vi "micron_update.vi"(0 "Position valid":bool, 2 "XYZ in":sgl[][](array[numeric])=[[-1290.5378, -2714.2402, -42.909184], [-1227.3542, -3608.3708, 102.94437]] format="%#.2f", 5 "Micron config":T12, 6 "error in":errorcluster, 8 "No pose":bool, 10 "Reset":bool, 11 "Trace index":i32, 16 "Parameters":T1={"Stimulus"={"Type"=enum."Off", "Phase"=0.0, "Amplitude"=[], "Injection point"=enum."Total pose", "Closed loop"=FALSE, "Offset"=[], "Tip -> world"=FALSE, "Frequency"=0.0, "Length"=0.0}, "Goal Filter A"={"Speedup max"=0.0, "Speedup thresh"=0.0, "Speedup nonlin"=0.0, "Filters"=[]}, "Mode controls"={"Hold"=FALSE, "Cancellation"=FALSE, "Goal filter"=FALSE, "Trigger"=FALSE}, "Manipulator type"=enum."Current piezo", "Manipulator calibration"={"Tool offsets"=[[0.0, 0.0, 36200.0]], "Handle light calibration"=[], "Base pivots"=[], "Output pivots"=[], "Length center"=0.0, "Workspace height"=[], "Workspace diameter"=[0.0, 0.0, 36200.0], "Stack travel"=400.0, "Saturation pos"=375.0, "Inverse filters"=[], "Strut length"=0.0, "Tip light calibration"=[]}, "Network"={"Remote Host"="", "Send Status"=FALSE, "Send Port"=0, "Recv Commands"=FALSE, "Recv Port"=0}, "Goal Filter B"={"Speedup max"=0.0, "Speedup thresh"=0.0, "Speedup nonlin"=0.0, "Filters"=[]}, "Cancellation"={"KP"={"XY"=0.0, "Rxy"=0.0, "Z"=0.0, "Rz"=0.0}, "KI"=0.0, "KD"={"XY"=0.0, "Rxy"=0.0, "Z"=0.0, "Rz"=0.0}, "Max vel"=20.0, "Max acc"=0.001, "Int error limit"=3.0, "RCM gain"=0.0, "Bypass"=FALSE, "Degraded gain"=0.0}, "Transition time"=0.0, "Estimation"={"Link"={"Measure noise"=[], "Process noise"=[], "Alt process noise"=[], "Alt turnoff cycles"=20, "Innovation limit"=[], "Residue threshold"=0.0, "Enable"=FALSE}, "Handle"={"Measure noise"=[], "Process noise"=[], "State limits"=[], "Innovation limit"=[], "Prediction Lookahead"=0.0, "Enable"=FALSE}}} {"Transition time" format="%_3f"; "Cancellation"."Degraded gain" min=0 max=1 step=0.1 format="%#_3p"; "Cancellation"."RCM gain" min=0 max=1 step=0.1 format="%#_3p"; "Cancellation"."KD"."Rz" min=-1 max=1 step=0.01 format="%#_3p"; "Cancellation"."KD"."Rxy" min=-1 max=1 step=0.01 format="%#_3p"; "Cancellation"."KD"."Z" min=-1 max=1 step=0.01 format="%#_3p"; "Cancellation"."KD"."XY" min=-1 max=1 step=0.01 format="%#_3p"; "Cancellation"."KI" min=0 max=1 step=0.01 format="%#_3p"; "Cancellation"."KP"."Rz" min=-1 max=1 step=0.01 format="%#_3p"; "Cancellation"."KP"."Rxy" min=-1 max=1 step=0.01 format="%#_3p"; "Cancellation"."KP"."Z" min=-1 max=1 step=0.01 format="%#_3p"; "Cancellation"."KP"."XY" min=-1 max=1 step=0.01 format="%#_3p"; "Cancellation"."Max acc" format="%#_3p"; "Goal Filter B"."Filters"."V limit range" format="%_3p"; "Goal Filter B"."Filters"."V limit" format="%_3p"; "Goal Filter B"."Filters"."Upper Q" format="%_3f"; "Goal Filter B"."Filters"."Upper Fc" format="%_3p"; "Goal Filter B"."Filters"."Lower Q" format="%_3f"; "Goal Filter B"."Filters"."Scale factor" format="%_3f"; "Goal Filter B"."Filters"."Lower Fc" format="%_3p"; "Goal Filter B"."Speedup nonlin" format="%_3p"; "Goal Filter B"."Speedup thresh" format="%_3p"; "Goal Filter B"."Speedup max" format="%_3p"; "Manipulator calibration"."Tip light calibration" format="%#.1f"; "Manipulator calibration"."Strut length" format="%#_4p"; "Manipulator calibration"."Saturation pos" format="%#.1f"; "Manipulator calibration"."Stack travel" format="%#.1f"; "Manipulator calibration"."Length center" format="%#_4p"; "Manipulator calibration"."Output pivots" format="%#_6f"; "Manipulator calibration"."Base pivots" format="%#_6f"; "Manipulator calibration"."Handle light calibration" format="%#.1f"; "Goal Filter A"."Filters"."V limit range" format="%_3p"; "Goal Filter A"."Filters"."V limit" format="%_3p"; "Goal Filter A"."Filters"."Upper Q" format="%_3f"; "Goal Filter A"."Filters"."Upper Fc" format="%_3p"; "Goal Filter A"."Filters"."Lower Q" format="%_3f"; "Goal Filter A"."Filters"."Scale factor" format="%_3f"; "Goal Filter A"."Filters"."Lower Fc" format="%_3p"; "Goal Filter A"."Speedup nonlin" format="%_3p"; "Goal Filter A"."Speedup thresh" format="%_3p"; "Goal Filter A"."Speedup max" format="%_3p"; "Stimulus"."Length" min=0.0 max=100.0 step=100.0 format="%#_4p"; "Stimulus"."Frequency" min=0.0 step=100.0 format="%#_4g"; "Stimulus"."Offset" format="%#_3p"; "Stimulus"."Amplitude" format="%#_3p"; "Stimulus"."Phase" min=-180.0 max=360.0 step=100.0 format="%#.2f"}) -> (17 "Timestamp":u64, 26 "error out":errorcluster)   [LabVIEW 2014]
uses:
  initialization/micron_config.ctl
  manipulator/squiggle/Host/i2c_interface.ctl
  manipulator/squiggle/Host/fpga_reference.ctl
  testing/Micron params.ctl
  testing/stimulus.ctl
  testing/injection_point.ctl
  filtering/goal_loop_parms.ctl
  testing/mode_conrols.ctl
  testing/manipulator_cal.ctl
  asap/labview/testing/probe_calibration.ctl
  host/network_params.ctl
  sq_control_params.ctl
  decoupled_gain.ctl
  estimation_controls.ctl
  <vilib>/Analysis/Matrix/Datatypes/RealMatrix.ctl
  initialization/micron_globals.vi
  <vilib>/Analysis/Matrix/Numeric/Conversions/Matrix To Array - RM.vi
  <vilib>/Analysis/Matrix/NI_Matrix.lvlib
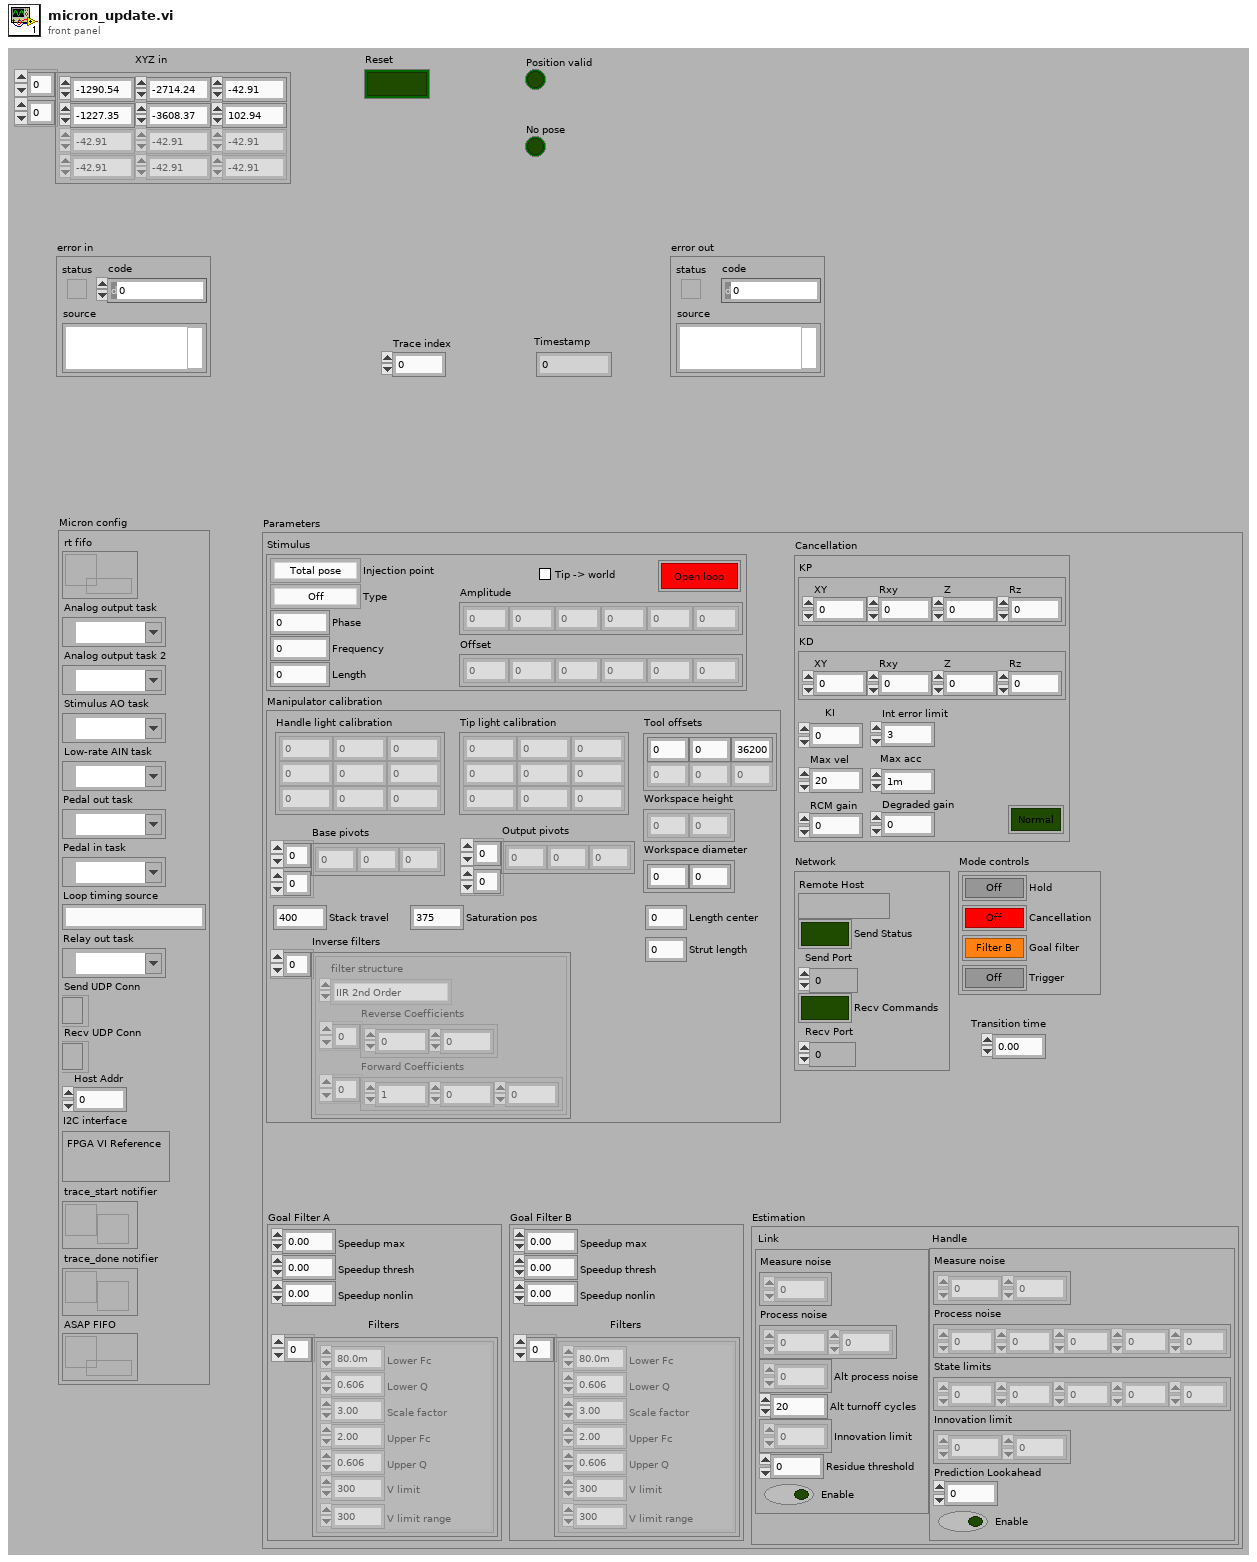
[diagram p1: front panel]
types:
  T1 = typedef "Micron params.ctl" = cluster{"Stimulus":T2, "Goal Filter A":T4, "Mode controls":T5, "Manipulator type":enum16{"Current piezo", "Voltage piezo"}, "Manipulator calibration":T6, "Network":T8, "Goal Filter B":T4, "Cancellation":T9, "Transition time":sgl, "Estimation":T11}
  T2 = typedef "stimulus.ctl" = cluster{"Type":enum16{"Off", "Step", "Sine", "Triangle", "Arbitrary"}, "Phase":dbl, "Amplitude":sgl[], "Injection point":T3, "Closed loop":bool, "Offset":sgl[], "Tip -> world":bool, "Frequency":dbl, "Length":dbl}
  T3 = typedef "injection_point.ctl" = enum16{"Total pose", "V limiter", "Goal ", "Link position", "KF link position", "Inverse kin", "Link goal", "Link error", "Controller", "Output", "Drive", "Light"}
  T4 = typedef "goal_loop_parms.ctl" = cluster{"Speedup max":sgl, "Speedup thresh":sgl, "Speedup nonlin":sgl, "Filters":cluster{"Lower Fc":sgl, "Lower Q":sgl, "Scale factor":sgl, "Upper Fc":sgl, "Upper Q":sgl, "V limit":sgl, "V limit range":sgl}[]}
  T5 = typedef "mode_conrols.ctl" = cluster{"Hold":bool, "Cancellation":bool, "Goal filter":bool, "Trigger":bool}
  T6 = typedef "manipulator_cal.ctl" = cluster{"Tool offsets":sgl[][], "Handle light calibration":T7, "Base pivots":sgl[][], "Output pivots":sgl[][], "Length center":sgl, "Workspace height":sgl[], "Workspace diameter":sgl[], "Stack travel":sgl, "Saturation pos":sgl, "Inverse filters":cluster{"filter structure":enum32{"IIR 2nd Order", "IIR 4th Order"}, "Reverse Coefficients":dbl[], "Forward Coefficients":dbl[]}[], "Strut length":sgl, "Tip light calibration":T7}
  T7 = typedef "probe_calibration.ctl" = sgl[][]
  T8 = typedef "network_params.ctl" = cluster{"Remote Host":string, "Send Status":bool, "Send Port":u16, "Recv Commands":bool, "Recv Port":u16}
  T9 = typedef "sq_control_params.ctl" = cluster{"KP":T10, "KI":sgl, "KD":T10, "Max vel":sgl, "Max acc":sgl, "Int error limit":sgl, "RCM gain":sgl, "Bypass":bool, "Degraded gain":sgl}
  T10 = typedef "decoupled_gain.ctl" = cluster{"XY":sgl, "Rxy":sgl, "Z":sgl, "Rz":sgl}
  T11 = typedef "estimation_controls.ctl" = cluster{"Link":cluster{"Measure noise":dbl[], "Process noise":dbl[], "Alt process noise":dbl[], "Alt turnoff cycles":i32, "Innovation limit":dbl[], "Residue threshold":dbl, "Enable":bool}, "Handle":cluster{"Measure noise":dbl[], "Process noise":dbl[], "State limits":dbl[], "Innovation limit":dbl[], "Prediction Lookahead":sgl, "Enable":bool}}
  T12 = typedef "micron_config.ctl" = cluster{"rt fifo":refnum<k33>, "Analog output task":refnum<k21>, "Analog output task 2":refnum<k21>, "Stimulus AO task":refnum<k21>, "Low-rate AIN task":refnum<k21>, "Pedal out task":refnum<k21>, "Pedal in task":refnum<k21>, "Loop timing source":string, "Relay out task":refnum<k21>, "Send UDP Conn":refnum<k16>, "Recv UDP Conn":refnum<k16>, "Host Addr":u32, "I2C interface":T13, "trace_start notifier":refnum<notifier>, "trace_done notifier":refnum<notifier>, "ASAP FIFO":refnum<k33>}
  T13 = typedef "i2c_interface.ctl" = cluster{"FPGA VI Reference":T14}
  T14 = typedef "fpga_reference.ctl" = refnum<k20>
  T15 = typedef "NI_Matrix.lvlib/RealMatrix.ctl" = dbl[][]
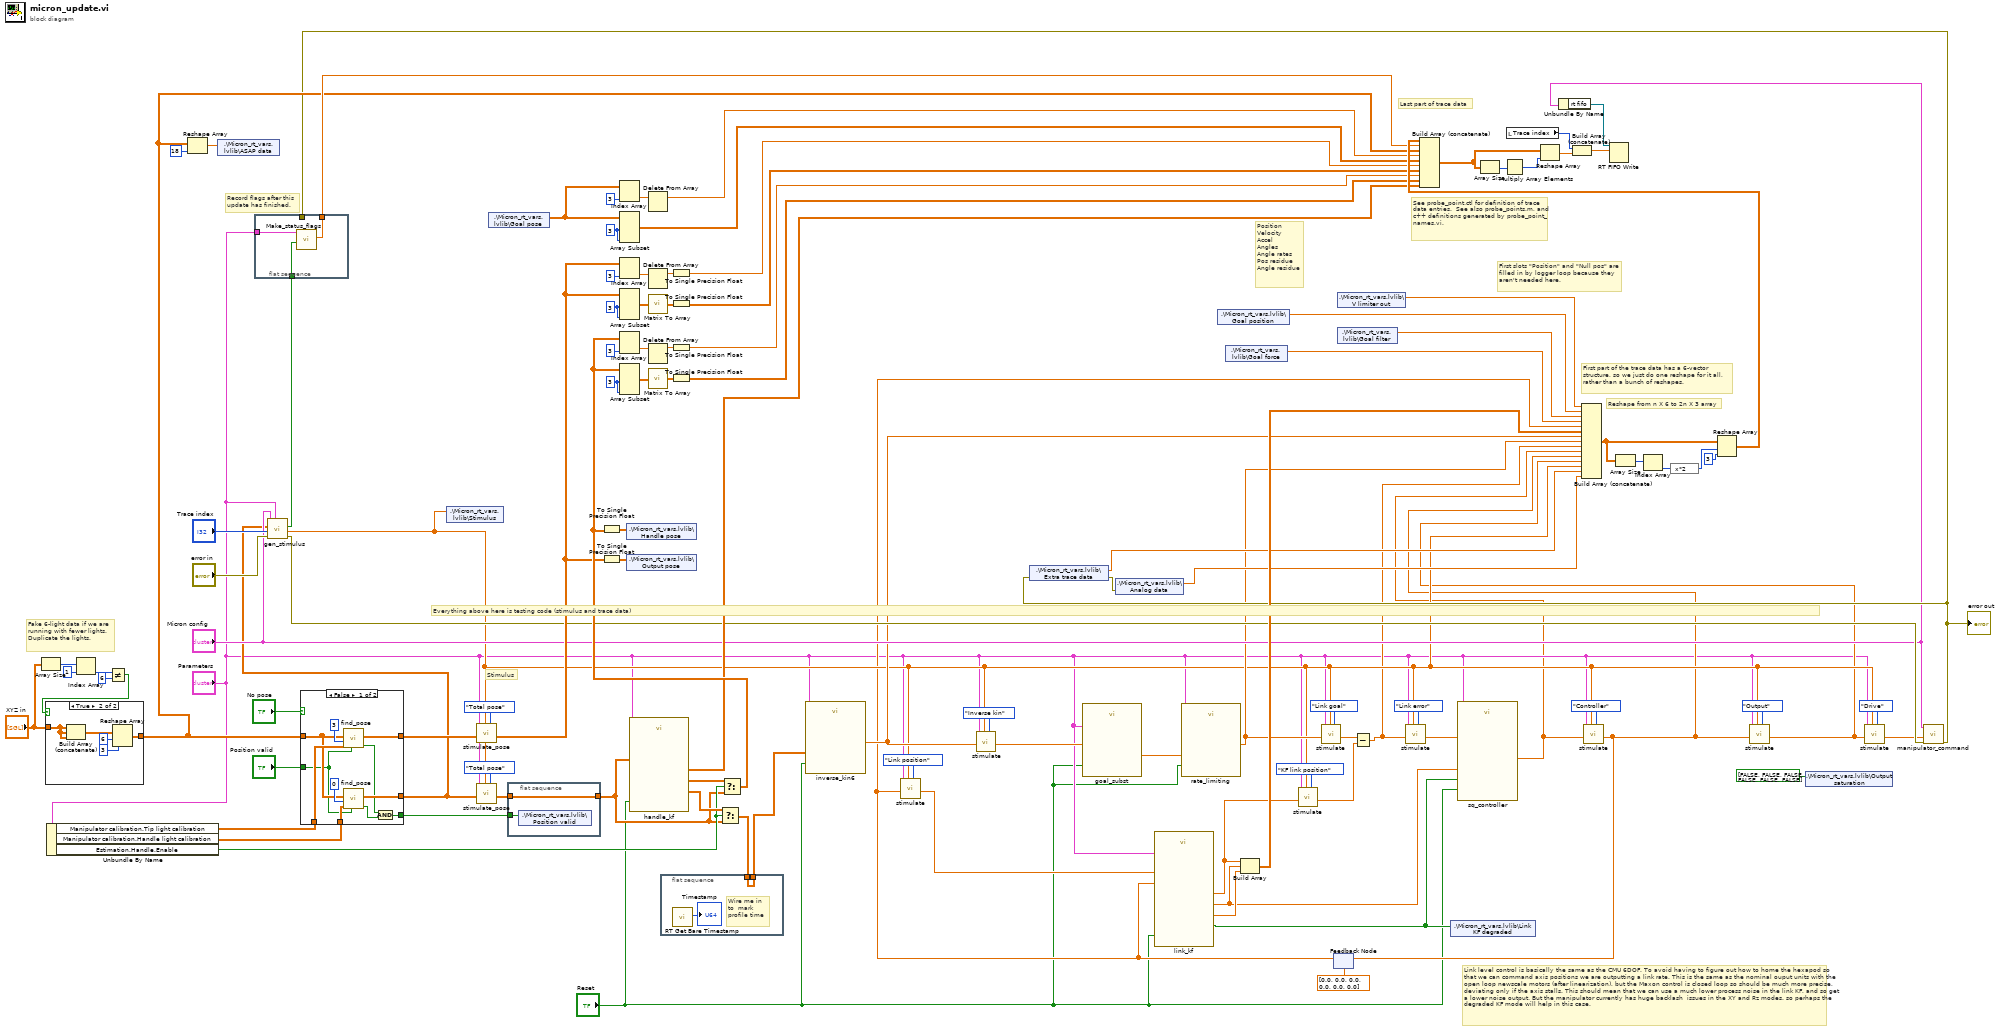
[diagram p0: block diagram]
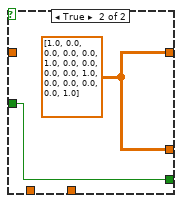
[diagram p2: hidden frame]
diagram:
  w73 = 3 ("length")
  w80 = 3 ("length")
  w107 = 3 ("length")
  # "Link level control is basically the same as the CMU 6DOF. To avoid having to figure out how to home the hexapod so that we can command axis positions we are outputting a link rate. This is the same as the nominal ouput units with the open loop newscale motors (after linearization), but the Maxon control is closed loop so should be much more precise, deviating only if the axis stalls. This should mean that we can use a much lower process noise in the link KF, and so get a lower noise output. But the manipulator currently has huge backlash  issues in the XY and Rz modes. so perhaps the degraded KF mode will help in this case."
  # "Position\nVelocity\nAccel\nAngles\nAngle rates\nPos residue\nAngle residue"
  # "Record flags after this\nupdate has finished."
  # "Fake 6-light data if we are running with fewer lights. Duplicate the lights."
  # "First slots \"Position\" and \"Null pos\" are filled in by logger loop because they aren't needed here."
  # "Last part of trace data"
  # "First part of the trace data has a 6-vector structure, so we just do one reshape for it all, rather than a bunch of reshapes."
  # "Reshape from n X 6 to 2n X 3 array"
  # "Everything above here is testing code (stimulus and trace data)"
  # "Stimulus"
  # "See probe_point.ctl for definition of trace data entries.  See also probe_points.m, and c++ definitions generated by probe_point_names.vi."
  n1 = Array Size(array="XYZ in") -> (size(s)=w51:i32[])
  n2 = Unbundle By Name("Parameters") -> ("Manipulator calibration.Tip light calibration"=w86:T7, "Manipulator calibration.Handle light calibration"=w67:T7, "Estimation.Handle.Enable"=w57:bool)
  n3 = Index Array(array=w51, index=1) -> (element=w49:i32)
  n4 = Not Equal?(x=w49, y=6) -> (x != y?=w47:bool)
  n5 = case shown="True" w47 {
    tunnel: [w112 w115] -> w64
    tunnel: "XYZ in" -> [w112 w113]
    frame False {
    }
    frame True {
      n6 = Build Array (concatenate)(w113, w113, w113) -> (w114:sgl[][])
      n7 = Reshape Array(w114, 6 ("dimension size"), 3 ("dimension size")) -> (w115:sgl[][])
    }
  }
  n8 = Reshape Array(w64, 18 ("dimension size")) -> (w101:sgl[])
  n9 = shared-variable ".\\Micron_rt_vars.lvlib\\ASAP data"(w101) -> ()  [unwired: 2 out]
  n10 = flat-sequence {
    tunnel: [w120] -> w88
    tunnel: w56 -> [w119]
    tunnel: "Parameters" -> [w118]
    tunnel: w44 -> [_]
    frame #0 {
      n11 = call "Make_status_flags.vi"("Stimulus increasing"=w119, "Parameters"=w118) -> ("Status flags"=w120:sgl[])  [unwired: 9 out]
    }
  }
  n12 = case shown="False" "No pose" {
    tunnel: w86 -> [w130 _]
    tunnel: w67 -> [w129 _]
    tunnel: w64 -> [w127 _]
    tunnel: [w126 w132] -> w63
    tunnel: [w125 w132] -> w30
    tunnel: "Position valid" -> [w124 w133]
    tunnel: [w121 w133] -> w17
    frame False {
      n13 = call "find_pose.vi"("Position valid"=w124, "Light positions"=w130, "XYZ index"=3, "XYZ in"=w127) -> ("Pose valid"=w123:bool, "Pose"=w126:T15)  [unwired: 1 in, 5 out]
      n14 = call "find_pose.vi"("Position valid"=w124, "Light positions"=w129, "XYZ index"=0, "XYZ in"=w127) -> ("Pose valid"=w122:bool, "Pose"=w125:T15)  [unwired: 1 in, 5 out]
      n15 = And(x=w123, y=w122) -> (x .and. y?=w121:bool)
    }
    frame True {
      w132 = T15 [[1.0, 0.0, 0.0, 0.0], [0.0, 1.0, 0.0, 0.0], [0.0, 0.0, 1.0, 0.0], [0.0, 0.0, 0.0, 1.0]] ("LR transform")
    }
  }
  n16 = call "gen_stimulus.vi"("Parameters"="Parameters", "error in"="error in", "Trace index"="Trace index", "Raw handle pose"=w30, "Micron config"="Micron config") -> ("error out"=w55:errorcluster, "Stimulus"=w22:sgl[], "Stimulus increasing"=w56:bool)  [unwired: 4 out]
  n17 = shared-variable ".\\Micron_rt_vars.lvlib\\Stimulus"(w22) -> ()  [unwired: 2 out]
  n18 = call "stimulate_pose.vi"("Injection point"=injection_point."Total pose", "Stimulus"=w22, "Pose in"=w63, "Parameters"="Parameters") -> ("Pose out"=w61:T15)  [unwired: 6 in]
  n19 = call "stimulate_pose.vi"("Injection point"=injection_point."Total pose", "Stimulus"=w22, "Pose in"=w30, "Parameters"="Parameters") -> ("Pose out"=w19:T15)  [unwired: 6 in]
  n20 = shared-variable ".\\Micron_rt_vars.lvlib\\Goal pose"() -> (w70:sgl[][])  [unwired: 2 out]
  n21 = flat-sequence {
    tunnel: [w135] -> w18
    tunnel: w19 -> [w135]
    tunnel: w17 -> [w134]
    frame #0 {
      n22 = shared-variable ".\\Micron_rt_vars.lvlib\\Position valid"(w134) -> ()  [unwired: 2 out]
    }
  }
  n23 = To Single Precision Float(number=w61) -> (single precision float=w102:sgl[][])
  n24 = Index Array(array=w70, index (col)=3 ("disabled index (col)")) -> (element=w72:sgl[])  [unwired: 1 in]
  n25 = Array Subset(array=w70, length (row)=w73, length (col)=w73) -> (w69:sgl[][])  [unwired: 2 in]
  n26 = Index Array(array=w61, index (col)=3 ("disabled index (col)")) -> (element=w99:dbl[])  [unwired: 1 in]
  n27 = Array Subset(array=w61, length (row)=w107, length (col)=w107) -> (w106:T15)  [unwired: 2 in]
  n28 = shared-variable ".\\Micron_rt_vars.lvlib\\Output pose"(w102) -> ()  [unwired: 2 out]
  n29 = call "handle_kf.vi"("Reset"="Reset", "Parameters"="Parameters", "Handle Pose"=w18) -> ("Handle State"=w65:sgl[][], "Predicted Handle Pose"=w58:T15, "Handle Pose (KF)"=w59:T15)  [unwired: 6 in]
  n30 = Delete From Array(array=w72) -> (array with subset deleted=w26:sgl[])  [unwired: 2 in, 1 out]
  n31 = Delete From Array(array=w99) -> (array with subset deleted=w97:dbl[])  [unwired: 2 in, 1 out]
  n32 = call-poly <vilib>:"Matrix To Array.vi"("Real Matrix"=w106) -> ("Real 2D Array"=w105:dbl[][])
  n33 = flat-sequence {
    tunnel: [w136] -> w53
    tunnel: w54 -> [w136]
    frame #0 {
      # "Wire me in to  mark profile time"
      n34 = call "RT Get Bare Timestamp.vi"() -> ("Timestamp"=→"Timestamp":u64)  [unwired: 11 out]
    }
  }
  n35 = To Single Precision Float(number=w97) -> (single precision float=w25:sgl[])
  n36 = To Single Precision Float(number=w105) -> (single precision float=w89:sgl[][])
  n37 = Select(t=w58, s=w57, f=w18) -> (s? t:f=w54:T15)
  n38 = Select(t=w59, s=w57, f=w18) -> (s? t:f=w66:T15)
  n39 = To Single Precision Float(number=w66) -> (single precision float=w76:sgl[][])
  n40 = Index Array(array=w66, index (col)=3 ("disabled index (col)")) -> (element=w83:dbl[])  [unwired: 1 in]
  n41 = Array Subset(array=w66, length (row)=w80, length (col)=w80) -> (w81:T15)  [unwired: 2 in]
  n42 = shared-variable ".\\Micron_rt_vars.lvlib\\Handle pose"(w76) -> ()  [unwired: 1 in, 1 out]
  n43 = Delete From Array(array=w83) -> (array with subset deleted=w85:dbl[])  [unwired: 2 in, 1 out]
  n44 = call-poly <vilib>:"Matrix To Array.vi"("Real Matrix"=w81) -> ("Real 2D Array"=w82:dbl[][])
  n45 = To Single Precision Float(number=w85) -> (single precision float=w79:sgl[])
  n46 = To Single Precision Float(number=w82) -> (single precision float=w78:sgl[][])
  n47 = call "inverse_kin6.vi"("Reset"="Reset", "Predicted \nHandle pose"=w53, "Parameters"="Parameters") -> ("Link goal"=w23:sgl[])  [unwired: 8 in]
  n48 = call "stimulate.vi"("Injection point"=injection_point."Inverse kin", "Stimulus"=w22, "Input"=w23, "Parameters"="Parameters") -> ("Output"=w21:sgl[])  [unwired: 1 in, 5 out]
  n49 = call "goal_subst.vi"("Reset"="Reset", "Parameters"="Parameters", "Link goal"=w21) -> ("Substituted goal"=w45:sgl[])  [unwired: 3 in, 5 out]
  n50 = call "rate_limiting.vi"("Reset"="Reset", "Parameters"="Parameters", "Link goal"=w45) -> ("Substituted goal"=w27:sgl[])  [unwired: 8 in]
  n51 = shared-variable ".\\Micron_rt_vars.lvlib\\Goal position"() -> (w87:sgl[])  [unwired: 2 out]
  n52 = shared-variable ".\\Micron_rt_vars.lvlib\\Goal force"() -> (w15:sgl[])  [unwired: 2 out]
  n53 = call "stimulate.vi"("Injection point"=injection_point."Link goal", "Stimulus"=w22, "Input"=w27, "Parameters"="Parameters") -> ("Output"=w9:sgl[])  [unwired: 1 in, 5 out]
  n54 = feedback #1(sgl[] [0.0, 0.0, 0.0, 0.0, 0.0, 0.0] ("Output")) -> (w10:sgl[])
  n55 = call "stimulate.vi"("Injection point"=injection_point."Link position", "Stimulus"=w22, "Input"=w10, "Parameters"="Parameters") -> ("Output"=w32:sgl[])  [unwired: 1 in, 5 out]
  n56 = call "link_kf.vi"("Reset"="Reset", "Parameters"="Parameters", "Last output command"=w10, "Raw link position"=w32) -> ("Position residue"=w34:sgl[], "Link rates"=w3:sgl[], "KF link position"=w33:sgl[], "Degraded"=w2:bool[])  [unwired: 4 in]
  n57 = Build Array(w33, w3, w34) -> (w111:sgl[][])
  n58 = call "stimulate.vi"("Injection point"=injection_point."KF link position", "Stimulus"=w22, "Input"=w33, "Parameters"="Parameters") -> ("Output"=w8:sgl[])  [unwired: 1 in, 5 out]
  n59 = shared-variable ".\\Micron_rt_vars.lvlib\\V limiter out"() -> (w95:sgl[])  [unwired: 2 out]
  n60 = shared-variable ".\\Micron_rt_vars.lvlib\\Goal filter"() -> (w16:sgl[])  [unwired: 2 out]
  n61 = Subtract(x=w9, y=w8) -> (x-y=w7:sgl[])
  n62 = call "stimulate.vi"("Injection point"=injection_point."Link error", "Stimulus"=w22, "Input"=w7, "Parameters"="Parameters") -> ("Output"=w5:sgl[])  [unwired: 1 in, 5 out]
  n63 = shared-variable ".\\Micron_rt_vars.lvlib\\Link KF degraded"(w2) -> ()  [unwired: 1 in, 1 out]
  n64 = call "sq_controller.vi"("Degraded"=w2, "Reset"="Reset", "Parameters"="Parameters", "Link rates"=w3, "Link length error"=w5) -> ("Motor commands"=w4:sgl[])  [unwired: 6 in]
  n65 = local read "Trace index"() -> (w35:i32)
  n66 = Unbundle By Name("Micron config") -> ("rt fifo"=w40:refnum<k33>)
  n67 = call "stimulate.vi"("Injection point"=injection_point."Controller", "Stimulus"=w22, "Input"=w4, "Parameters"="Parameters") -> ("Output"=w13:sgl[])  [unwired: 1 in, 5 out]
  n68 = feedback-in #1(w13) -> ()
  n69 = call "stimulate.vi"("Injection point"=injection_point."Output", "Stimulus"=w22, "Input"=w13, "Parameters"="Parameters") -> ("Output"=w12:sgl[])  [unwired: 1 in, 5 out]
  n70 = shared-variable ".\\Micron_rt_vars.lvlib\\Output saturation"(bool[] [FALSE, FALSE, FALSE, FALSE, FALSE, FALSE] ("Degraded")) -> ()  [unwired: 2 out]
  n71 = call "stimulate.vi"("Injection point"=injection_point."Drive", "Stimulus"=w22, "Input"=w12, "Parameters"="Parameters") -> ("Output"=w46:sgl[])  [unwired: 1 in, 5 out]
  n72 = call "manipulator_command.vi"("Error in"=w55, "Manipulator command"=w46, "Micron config"="Micron config") -> ("Error out"=w44:errorcluster)  [unwired: 8 in]
  "error out" <- w44
  n73 = shared-variable ".\\Micron_rt_vars.lvlib\\Extra trace data"(error in=w44) -> (w110:sgl[], error out=w29:errorcluster)
  n74 = shared-variable ".\\Micron_rt_vars.lvlib\\Analog data"(error in=w29) -> (w28:sgl[])  [unwired: 1 out]
  n75 = Build Array (concatenate)(w95, w87, w16, w15, w10, w111, w23, w27, w7, w4, w13, w12, w22, w110, w28) -> (w90:sgl[][])
  n76 = Array Size(array=w90) -> (size(s)=w94:i32[])
  n77 = Index Array(array=w94) -> (element=w93:i32)  [unwired: 1 in]
  n78 = expression code="x*2"(w93) -> (w92:i32)
  n79 = Reshape Array(w90, w92, 3 ("dimension size")) -> (w109:sgl[][])
  n80 = Build Array (concatenate)(w109, w88, w64, w26, w69, w25, w89, w79, w78, w65) -> (w39:sgl[][])
  n81 = Array Size(array=w39) -> (size(s)=w38:i32[])
  n82 = Multiply Array Elements(1:w38) -> (0:w37:i32)
  n83 = Reshape Array(w39, w37) -> (w41:sgl[])
  n84 = Build Array (concatenate)(w35, w41) -> (w42:sgl[])
  n85 = RT FIFO Write(0:w40, 1:w42) -> ()  [unwired: 2 in, 5 out]
